vi "Car Main.vi"() -> ()   [LabVIEW 2015]
uses:
  <vilib>/Platform/TimedLoop/XDataNode/timing_clust.ctl
  <vilib>/Platform/TimedLoop/XDataNode/nitl_modes.ctl
  <vilib>/Platform/TimedLoop/XDataNode/wakeup.ctl
  <vilib>/FPGAPlugInAG/sbRIO-9627/niLvFpga_Open_sbRIO-9627.vi
  <vilib>/FPGAPlugInAG/sbRIO-9627/niLvFpga_Reset_sbRIO-9627.vi
  Global Data.vi
  <vilib>/Utility/error.llb/Error Cluster From Error Code.vi
  <vilib>/rvi/errors/niLvFpgaAdjustHostInterfaceError.vi
  <vilib>/FPGAPlugInAG/sbRIO-9627/niLvFpga_Close_sbRIO-9627.vi
  <vilib>/rvi/interface/nirviOpenFPGA/nirviOpenFPGA.xnode
  FPGA Bitfiles/Latest.lvbitx
  <vilib>/rvi/interface/nirviMethod/nirviMethod.xnode
  FPGA Typedef.ctl
  <vilib>/Platform/TimedLoop/XDataNode/XDataNode.xnode
  <vilib>/rvi/interface/nirviReadWriteControl/nirviReadWriteControl.xnode
  <vilib>/rvi/interface/nirviCloseFPGA/nirviCloseFPGA.xnode
  <vilib>/NI_Real-Time Target Support.lvlib
  <vilib>/Platform/TimedLoop/XDataNode/XDNodeRunTimeDep.lvlib
  NiFpgaLv.dll
panel:
  in  "baud rate (125000 bps)":u32=500000
  in  "Shutdown":bool
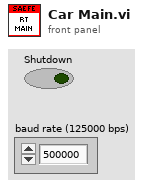
[diagram p1: front panel]
types:
  T1 = typedef "XDNodeRunTimeDep.lvlib/timing_clust.ctl" = cluster{"Expected End [f-1]":u64, "Actual End [f-1]":u64, "Finished Late? [f-1]":bool, "Expected End [i-1]":u64, "Actual End [i-1]":u64, "Finished Late? [i-1]":bool, "Expected Start [i]":u64, "Actual Start [i]":u64, "Expected Start [f]":u64, "Actual Start [f]":u64, "Source Name":string, "Structure Name":string, "Period":i64, "Deadline":i64, "Offset":i64, "Start":i64, "Priority":i32, "Timeout":i32, "Mode":T2, "Wakeup Reason":T3, "Error":errorcluster, "Source Type":string, "Secondary Source Type":string, "Global End Time":u64, "Global Start Time":u64, "Frame Duration":u64, "Iteration Duration":u64, "Assigned CPU":i32, "I/O Scan Engine Mode":u32}
  T2 = typedef "XDNodeRunTimeDep.lvlib/nitl_modes.ctl" = enum32{"No Change", "Process missed periods, maintain original phase", "Discard missed periods, maintain original phase", "Process missed periods, ignore original phase", "Discard missed periods, ignore original phase"}
  T3 = typedef "XDNodeRunTimeDep.lvlib/wakeup.ctl" = enum32{"Normal", "Aborted", "Asynchronous wakeup", "Timing source error", "Timed loop error", "Timeout"}
  T4 = typedef "CAN Message Queue.ctl" = refnum<k33>
  T5 = typedef "FPGA Typedef.ctl" = refnum<k20>
  T6 = typedef "Remote Stop Type.ctl" = cluster{"bRemoteStop":bool, "bRemoteEmergencyStop":bool, "bRemoteReturnToPits":bool, "bRemoteNewLogs":bool}
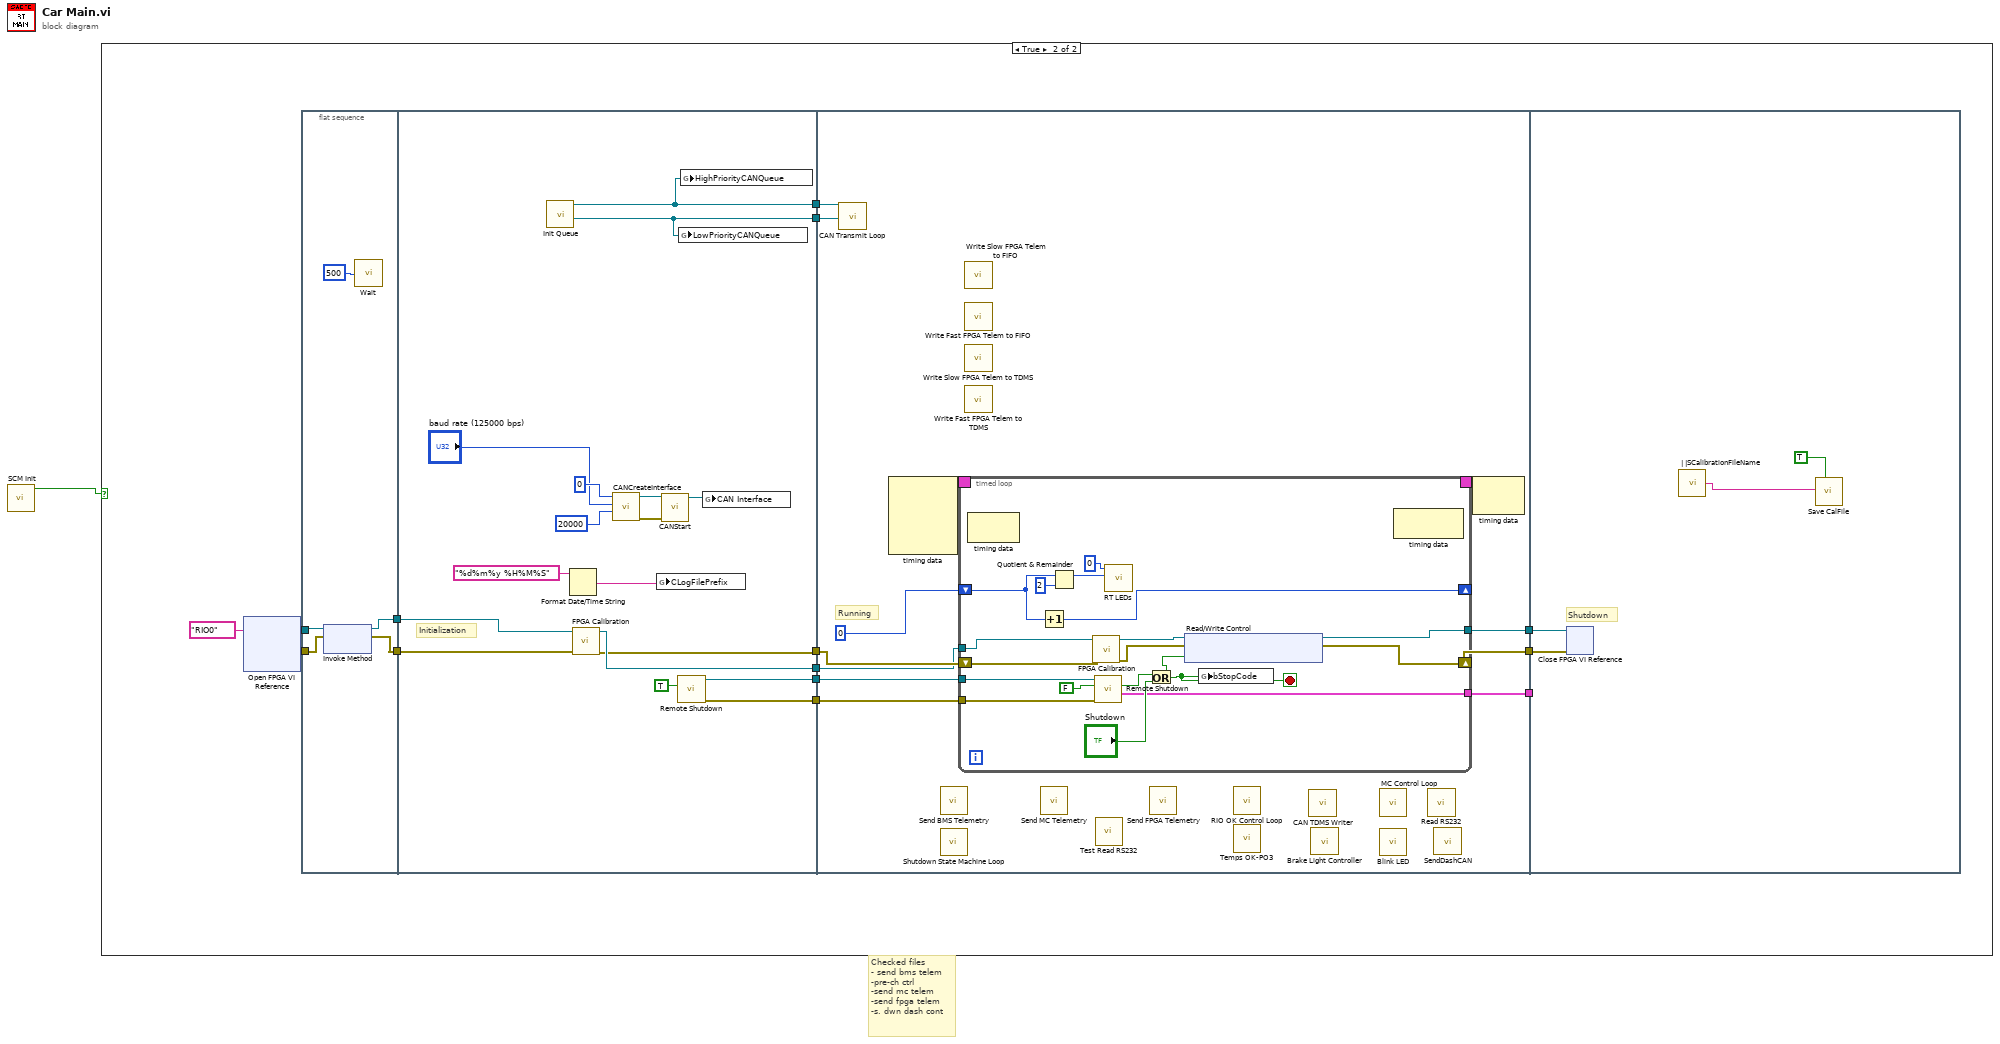
[diagram p0: block diagram]
diagram:
  # "Checked files\n- send bms telem\n-pre-ch ctrl\n-send mc telem\n-send fpga telem\n-s. dwn dash cont"
  n1 = call "SCM Init"() -> ("InitOK"=w1:bool)  [unwired: 3 in, 2 out]
  n2 = case shown="True" w1 {
    frame False {
    }
    frame True {
      n3 = xnode "Open FPGA VI Reference"("resource name"=tag "RIO0") -> ("FPGA VI Reference Out"=w4:refnum<k20>, "error out"=w3:errorcluster)  [unwired: 1 in]
      n4 = flat-sequence {
        tunnel: w3 -> [w18]
        tunnel: w4 -> [w19]
        tunnel: [w17] -> w15
        tunnel: [w16] -> w14
        tunnel: [w25] -> w13
        tunnel: [w24] -> w12
        tunnel: [w36] -> w11
        tunnel: [w35] -> w10
        tunnel: w15 -> [w26]
        tunnel: w14 -> [w23]
        tunnel: [w22] -> w9
        tunnel: [w21] -> w8
        tunnel: w13 -> [w38]
        tunnel: w12 -> [w39]
        tunnel: w11 -> [w48]
        tunnel: w10 -> [w47]
        tunnel: [w46] -> w7
        tunnel: [w43] -> w6
        tunnel: [w42] -> w5
        tunnel: w9 -> [w41]
        tunnel: w8 -> [w40]
        tunnel: w7 -> [_]
        tunnel: w6 -> [w75]
        tunnel: w5 -> [w74]
        frame #0 {
          n5 = xnode "Invoke Method"("FPGA VI Reference In"=w19, "error in"=w18) -> ("FPGA VI Reference Out"=w16:refnum<k20>, "error out"=w17:errorcluster)
          n6 = call "Wait"("Count(mSec)"=u32 500) -> ()  [unwired: 1 out]
        }
        frame #1 {
          # "Initialization"
          n7 = call "Init Queue.vi"() -> ("LowPriorityQueue"=w21:T4, "HighPriorityQueue"=w22:T4)  [unwired: 10 in]
          n8 = Format Date/Time String(time format string (%c)="%d%m%y %H%M%S") -> (date/time string=w27:string)  [unwired: 2 in]
          n9 = call "FPGA Calibration.vi"("error in"=w26, "FPGA Interface"=w23) -> ("error out"=w24:errorcluster, "FPGA Interface 2"=w25:T5)  [unwired: 8 in]
          n10 = call <vilib>:"CANCreateInterface.vi"("receive queue size (5)"=u32 20000, "baud rate (125000 bps)"="baud rate (125000 bps)", "interface index"=u32 0) -> ("error out"=w32:errorcluster, "interface object out"=w31:refnum<k20>)  [unwired: 7 in]
          n11 = global write "Global Data.vi" "CLogFilePrefix"(w27) -> ()
          n12 = call <vilib>:"CANStart.vi"("error in (no error)"=w32, "interface object in"=w31) -> ("interface object out"=w29:refnum<k20>)  [unwired: 8 in, 1 out]
          n13 = call "Remote Shutdown.vi"("Init?"=TRUE) -> ("error out 2"=w35:errorcluster, "port 2"=w36:refnum<k16>)  [unwired: 7 in, 2 out]
          n14 = global write "Global Data.vi" "LowPriorityCANQueue"(w21) -> ()
          n15 = global write "Global Data.vi" "HighPriorityCANQueue"(w22) -> ()
          n16 = global write "Global Data.vi" "CAN Interface"(w29) -> ()
        }
        frame #2 {
          # "Running"
          n17 = call "CAN Transmit Loop.vi"("LowPriorityQueue"=w40, "HighPriorityQueue"=w41) -> ()  [unwired: 10 in]
          n18 = node-c288() -> (w45:T1)  [unwired: 4 in]
          n19 = call "Send BMS Telemetry.vi"() -> ()  [unwired: 12 in]
          n20 = call "Shutdown State Machine Loop.vi"() -> ()  [unwired: 12 in]
          n21 = timed-loop {
            tunnel: w38 -> [w53]
            shift-right: [w63] -> _
            shift-left: 0 ("LED Num") -> [w62]
            tunnel: w48 -> [w59]
            tunnel: w47 -> [w58]
            tunnel: [w56] -> w46
            timing: w45 -> [_]
            timing-out: [_] -> w44
            tunnel: [w55] -> w43
            shift-right: [w54] -> w42
            shift-left: w39 -> [w52]
            stop <- w67 stop-if-true
            n22 = node-c288() -> ()  [unwired: 1 in, 1 out]
            n23 = Increment(x=w62) -> (x+1=w63:i32)
            n24 = Quotient & Remainder(x=w62, y=2) -> (x-y*floor(x/y)=w60:i32)  [unwired: 1 out]
            n25 = call "FPGA Calibration.vi"("error in"=w52, "FPGA Interface"=w53) -> ("error out"=w50:errorcluster, "FPGA Interface 2"=w51:T5)  [unwired: 8 in]
            n26 = call "Remote Shutdown.vi"("error out"=w58, "Init?"=FALSE, "port"=w59) -> ("REMOTE STOP"=w56:T6, "Shutdown?"=w65:bool)  [unwired: 5 in, 2 out]
            n27 = call <vilib>:"RT LEDs.vi"("State"=w60, "LED Num"=0) -> ()  [unwired: 4 in, 2 out]
            n28 = Or(x=w65, y="Shutdown") -> (x .or. y?=w67:bool)
            n29 = xnode "Read/Write Control"("FPGA VI Reference In"=w51, "error in"=w50, "stop"=w67) -> ("FPGA VI Reference Out"=w55:T5, "error out"=w54:errorcluster)
            n30 = global write "Global Data.vi" "bStopCode"(w67) -> ()
            n31 = node-c288() -> ()  [unwired: 1 in, 1 out]
          }
          n32 = call "Write Slow FPGA Telem to FIFO.vi"() -> ()  [unwired: 12 in]
          n33 = call "Write Fast FPGA Telem to FIFO.vi"() -> ()  [unwired: 12 in]
          n34 = call "Write Slow FPGA Telem to TDMS.vi"() -> ()  [unwired: 12 in]
          n35 = call "Write Fast FPGA Telem to TDMS.vi"() -> ()  [unwired: 12 in]
          n36 = call "Send MC Telemetry.vi"() -> ()  [unwired: 12 in]
          n37 = call "Test Read RS232.vi"() -> ()  [unwired: 12 in]
          n38 = call "Send FPGA Telemetry.vi"() -> ()  [unwired: 12 in]
          n39 = call "RIO OK Control Loop.vi"() -> ()  [unwired: 12 in]
          n40 = call "Temps OK-PO3.vi"() -> ()  [unwired: 12 in]
          n41 = call "CAN TDMS Writer.vi"() -> ()  [unwired: 12 in]
          n42 = call "Brake Light Controller.vi"() -> ()  [unwired: 12 in]
          n43 = call "MC Control Loop.vi"() -> ()  [unwired: 12 in]
          n44 = call "Blink LED.vi"() -> ()  [unwired: 12 in]
          n45 = call "Read RS232.vi"() -> ()  [unwired: 12 in]
          n46 = call "SendDashCAN.vi"() -> ()  [unwired: 12 in]
          n47 = node-c288(w44) -> ()  [unwired: 1 out]
        }
        frame #3 {
          # "Shutdown"
          n48 = xnode "Close FPGA VI Reference"("FPGA VI Reference In"=w75, "error in"=w74) -> ()  [unwired: 1 out]
          n49 = call "| |SCalibrationFileName"() -> ("Value"=w72:string)
          n50 = call <vilib>:"Save CalFile.vi"("Controls Only (F)"=TRUE, "Calibration File"=w72) -> ()  [unwired: 9 in, 1 out]
        }
      }
    }
  }
